vi "Write Numeric Parameters to string.vi"(1 "Parameters - numeric":T1[](array[typedef])) -> (0 "String":string)   [LabVIEW 2020, in "Run Utilities.lvlib" / "Optimiser Cell.lvclass"]
uses:
  Optimiser Cell.lvclass
  Optimise parameter - numeric.ctl
  Optimiser Cell.lvclass/Optimiser Cell.ctl
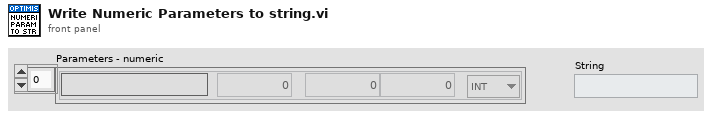
[diagram p1: front panel]
types:
  T1 = typedef "Run Utilities.lvlib/Optimiser Cell.lvclass/Optimise parameter - numeric.ctl" = cluster{"Name":string, "Start value":dbl, "From":dbl, "To":dbl, "dtype":enum16{"INT", "DBL"}}
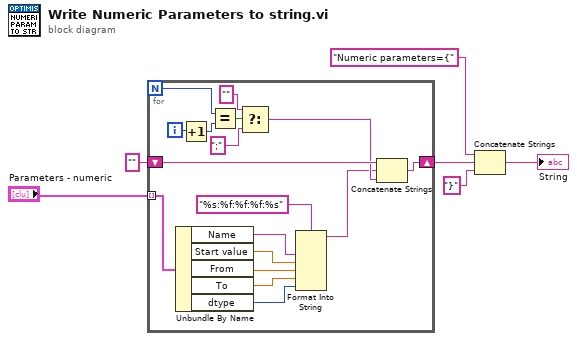
[diagram p0: block diagram]
diagram:
  n1 = for {
    N -> [w19]
    shift-right: [w22] -> w2
    shift-left: "" -> [w23]
    tunnel: "Parameters - numeric" -> [w7] mode=indexing
    i -> [w21]
    n2 = Unbundle By Name(w7) -> ("Name"=w14:string, "Start value"=w13:dbl, "From"=w12:dbl, "To"=w11:dbl, "dtype"=w10:enum16{"INT", "DBL"})
    n3 = Increment(x=w21) -> (x+1=w20:i32)
    n4 = Equal?(x=w19, y=w20) -> (x = y?=w18:bool)
    n5 = Select(t="" ("string"), s=w18, f=";") -> (s? t:f=w15:string)
    n6 = Format Into String(format string="%s:%f:%f:%f:%s", w14, w13, w12, w11, w10) -> (resulting string=w8:string)  [unwired: 2 in, 1 out]
    n7 = Concatenate Strings(w23, w8, w15) -> (w22:string)
  }
  n8 = Concatenate Strings("Numeric parameters={" ("string"), w2, "}" ("string")) -> (→"String":string)
